vi "PPCS_Vision_Get_Pose.vi"() -> (1 "Vison Pose":T1={"TRANSLATION"={"X"=0.0, "Y"=0.0}, "ROTATION"={"VALUE"=0.0, "COS"=1.0, "SIN"=0.0}} {"ROTATION"."SIN" format="%13.4f"; "ROTATION"."COS" format="%13.4f"; "ROTATION"."VALUE" format="%13.4f"; "TRANSLATION"."Y" format="%14.3f"; "TRANSLATION"."X" format="%14.3f"}, 3 "Have Vision Pose":bool)   [LabVIEW 2019]
uses:
  <vilib>/Rock Robotics/WPI/ThirdParty/JAS_Junk/TrajLib/TypeDef/POSE2D.ctl
  <vilib>/Rock Robotics/WPI/ThirdParty/JAS_Junk/TrajLib/TypeDef/TRANSLATION2D.ctl
  <vilib>/Rock Robotics/WPI/ThirdParty/JAS_Junk/TrajLib/TypeDef/ROTATION2D.ctl
  <vilib>/Rock Robotics/WPI/ThirdParty/JAS_Junk/TrajLib/VI/numCmd_ObtainQueue_Generic.vi
  PPCS_Vision_Globals.vi
  <vilib>/Rock Robotics/WPI/ThirdParty/JAS_Junk/TrajLib/Trajectory_Library.lvlib
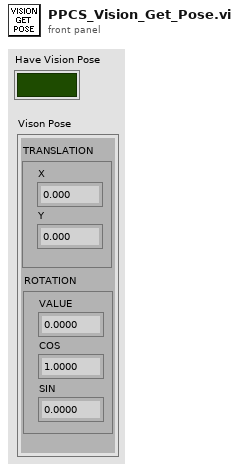
[diagram p1: front panel]
types:
  T1 = typedef "Trajectory_Library.lvlib/POSE2D.ctl" = cluster{"TRANSLATION":T2, "ROTATION":T3}
  T2 = typedef "Trajectory_Library.lvlib/TRANSLATION2D.ctl" = cluster{"X":dbl, "Y":dbl}
  T3 = typedef "Trajectory_Library.lvlib/ROTATION2D.ctl" = cluster{"VALUE":dbl, "COS":dbl, "SIN":dbl}
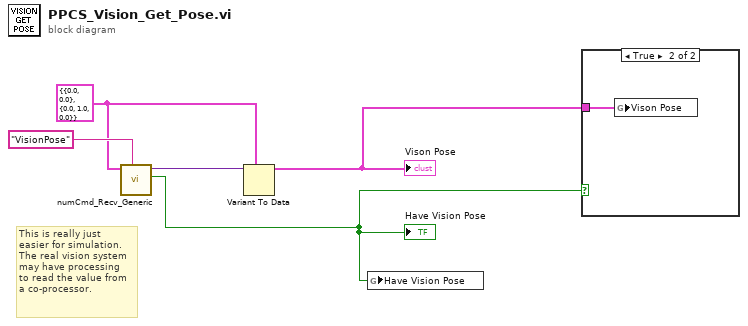
[diagram p0: block diagram]
diagram:
  w1 = T1 {"TRANSLATION"={"X"=0.0, "Y"=0.0}, "ROTATION"={"VALUE"=0.0, "COS"=1.0, "SIN"=0.0}} ("Vison Pose")
  # "This is really just\neasier for simulation.\nThe real vision system\nmay have processing\nto read the value from\na co-processor."
  n1 = call <vilib>:"numCmd_Recv_Generic.vi"("Command Name"="VisionPose", "Initial Value"=w1) -> ("Changed"=w3:bool, "Newest Value"=w5:variant)  [unwired: 7 in, 1 out]
  "Have Vision Pose" <- w3
  n2 = Variant To Data(type=w1, Variant=w5) -> (data=w2:T1)  [unwired: 1 in, 1 out]
  "Vison Pose" <- w2
  n3 = global write "PPCS_Vision_Globals.vi" "Have Vision Pose"(w3) -> ()
  n4 = case shown="True" w3 {
    tunnel: w2 -> [_ w6]
    frame False {
    }
    frame True {
      n5 = global write "PPCS_Vision_Globals.vi" "Vison Pose"(w6) -> ()
    }
  }
